vi "swmm_stop.vi"(4 "error in":errorcluster, 7 "Success msg?":bool) -> (0 "error out":errorcluster, 1 "qual error":dbl, 2 "flow error":dbl, 3 "runoff error":dbl)   [LabVIEW 2014]
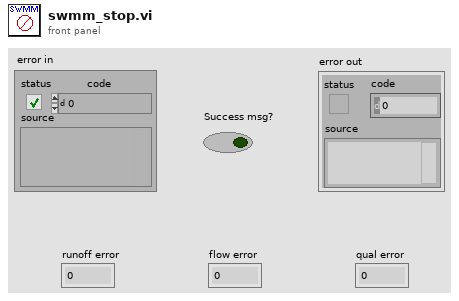
[diagram p1: front panel]
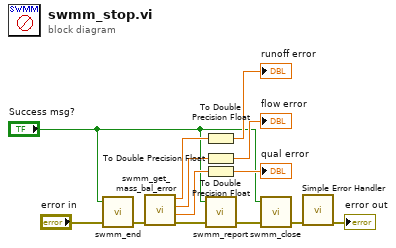
[diagram p0: block diagram]
diagram:
  n1 = call "swmm_end.vi"("error in (no error)"="error in", "Success msg?"="Success msg?") -> ("error out"=w13:errorcluster)  [unwired: 3 in]
  n2 = call "swmm_get_mass_bal_error.vi"("error in (no error)"=w13) -> ("error out"=w12:errorcluster, "qual_error"=w3:sgl, "flow_error"=w4:sgl, "runoff_error"=w8:sgl)  [unwired: 5 in]
  n3 = To Double Precision Float(number=w8) -> (double precision float=→"runoff error":dbl)
  n4 = To Double Precision Float(number=w4) -> (double precision float=→"flow error":dbl)
  n5 = To Double Precision Float(number=w3) -> (double precision float=→"qual error":dbl)
  n6 = call "swmm_report.vi"("error in (no error)"=w12, "Show success msg?"="Success msg?") -> ("error out"=w1:errorcluster)  [unwired: 3 in]
  n7 = call "swmm_close.vi"("error in (no error)"=w1, "Success msg?"="Success msg?") -> ("error out"=w11:errorcluster)  [unwired: 3 in]
  n8 = call <vilib>:"Simple Error Handler.vi"("error in (no error)"=w11) -> ("error out"=→"error out":errorcluster)  [unwired: 4 in, 4 out]
